vi "CatapultLightSensorControl.vi"   [LabVIEW 2015]
uses:
  Utilities/MotorPositionGlobals.vi
types:
  T1 = typedef "WPI_SwitchDevRef.ctl" = cluster{"DevStatus":errorcluster, "DIO Channel":T2, "CntIndex":T3, "Normally Closed":bool}
  T2 = typedef "FPGA_DIOChannel.ctl" = enum8{"DIO 0", "DIO 1", "DIO 2", "DIO 3", "DIO 4", "DIO 5", "DIO 6", "DIO 7", "DIO 8", "DIO 9", "DIO MXP 0", "DIO MXP 1", "DIO MXP 2", "DIO MXP 3", "DIO MXP 4", "DIO MXP 5", "DIO MXP 6", "DIO MXP 7", "DIO MXP 8", "DIO MXP 9", "DIO MXP 10", "DIO MXP 11", "DIO MXP 12", "DIO MXP 13", "DIO MXP 14", "DIO MXP 15", "Invalid"}
  T3 = typedef "FPGA_CounterCtrSystemIndex.ctl" = enum8{"Ctr 0", "Ctr 1", "Ctr 2", "Ctr 3", "Ctr 4", "Ctr 5", "Ctr 6", "Ctr 7", "Invalid"}
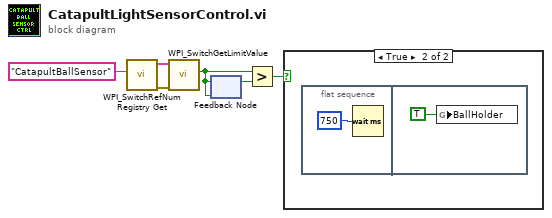
[diagram p0: block diagram]
diagram:
  n1 = call <vilib>:"WPI_SwitchRefNum Registry Get.vi"("refnum name"="CatapultBallSensor") -> ("error out"=w6:errorcluster, "SwitchDevRef"=w5:T1)  [unwired: 9 in]
  n2 = call <vilib>:"WPI_SwitchGetLimitValue.vi"("error in (no error)"=w6, "SwitchDevRef"=w5) -> ("Switch Pressed"=w3:bool)  [unwired: 7 in, 2 out]
  n3 = feedback-in #1(w3) -> ()
  n4 = feedback #1(w3) -> (w2:bool)
  n5 = Greater?(x=w3, y=w2) -> (0:w1:bool)
  n6 = case shown="True" w1 {
    frame False {
    }
    frame True {
      n7 = flat-sequence {
        frame #0 {
          n8 = Wait (ms)(milliseconds to wait=u32 750) -> ()  [unwired: 1 out]
        }
        frame #1 {
          n9 = global write "MotorPositionGlobals.vi" "BallHolder"(TRUE ("BallHolder")) -> ()
        }
      }
    }
  }
